vi "Startup.vi"(8 "error in (no error)":errorcluster, 11 "Data Cluster In":T1={"Status"="", "SQLite"=refnum, "StationConfig"={"station_id"="", "schema_version"="", "sqlite_path"="", "syncagent_db_path"="", "postgres_conn"="", "sync_interval_sec"=0, "inbound_offset_sec"=0, "batch_size"=0, "table_overrides"=[]}, "OB Module ID"=-1, "IB Module ID"=-1, "is online"=FALSE, "CM alive?"=FALSE, "OB alive?"=FALSE, "IB alive?"=FALSE, "IB first cycle seen?"=FALSE, "OB first cycle seen?"=FALSE, "shutting down?"=FALSE, "exit code"=0, "status"=FALSE, "code"=0, "source"="", "ShutdownReason"=enum."None", "OB last cycle at"=timestamp(0 s since 1904-01-01), "IB last cycle at"=timestamp(0 s since 1904-01-01), "Baseline Config"={"Baseline Mode"=enum."None", "From Date"="", "Chunk Size"=1000, "Verify Checksums"=TRUE}}) -> (0 "error out":errorcluster, 1 "halt?":bool, 3 "Data Cluster Out":T1={"Status"="", "SQLite"=refnum, "StationConfig"={"station_id"="", "schema_version"="", "sqlite_path"="", "syncagent_db_path"="", "postgres_conn"="", "sync_interval_sec"=0, "inbound_offset_sec"=0, "batch_size"=0, "table_overrides"=[]}, "OB Module ID"=-1, "IB Module ID"=-1, "is online"=FALSE, "CM alive?"=FALSE, "OB alive?"=FALSE, "IB alive?"=FALSE, "IB first cycle seen?"=FALSE, "OB first cycle seen?"=FALSE, "shutting down?"=FALSE, "exit code"=0, "status"=FALSE, "code"=0, "source"="", "ShutdownReason"=enum."None", "OB last cycle at"=timestamp(0 s since 1904-01-01), "IB last cycle at"=timestamp(0 s since 1904-01-01), "Baseline Config"={"Baseline Mode"=enum."None", "From Date"="", "Chunk Size"=1000, "Verify Checksums"=TRUE}})   [LabVIEW 2025, in "Dashboard.lvlib"]
uses:
  Dashboard.lvlib
  OpCore/SQLite/SQLite.lvclass
  OpCore/PostgreSQL/PostgreSQL.lvclass
  OpCore/Baseline/Baseline.lvclass
  OpCore/OpCore Foundation/OpCore Foundation.lvlib
  OpCore/OpCore Types/SyncCycleResult.ctl
  OpCore/OpCore Types/OpCore Types.lvlib
  OpCore/OpCore Types/CycleStatus.ctl
  OpCore/OpCore Types/CycleDirection.ctl
  OpCore/OpCore Types/SyncDirection.ctl
  OpCore/OpCore Types/TableOverride.ctl
  OpCore/OpCore Types/StationConfig.ctl
  OpCore/OpCore Types/ShutdownReason.ctl
  OpCore/OpCore Types/BaselineMode.ctl
  OpCore/OpCore Types/Baseline Config.ctl
  Module Data--cluster.ctl
panel:
  # "C:\\Works\\OpCore\\Data\\station-01.db"
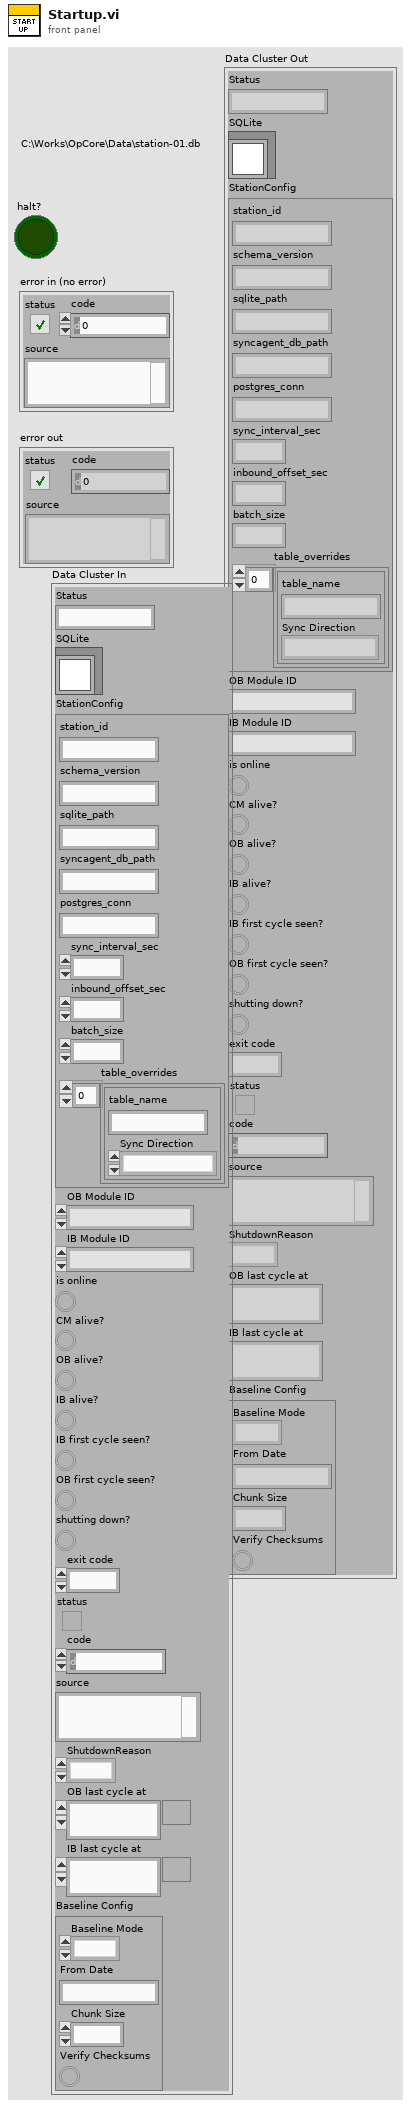
[diagram p1: front panel]
types:
  T1 = typedef "Dashboard.lvlib/Module Data--cluster.ctl" = cluster{"Status":string, "SQLite":refnum<class "SQLite.lvclass">, "StationConfig":T2, "OB Module ID":i32, "IB Module ID":i32, "is online":bool, "CM alive?":bool, "OB alive?":bool, "IB alive?":bool, "IB first cycle seen?":bool, "OB first cycle seen?":bool, "shutting down?":bool, "exit code":i32, "status":bool, "code":i32, "source":string, "ShutdownReason":T5, "OB last cycle at":timestamp, "IB last cycle at":timestamp, "Baseline Config":T6}
  T2 = typedef "OpCore Types.lvlib/StationConfig.ctl" = cluster{"station_id":string, "schema_version":string, "sqlite_path":string, "syncagent_db_path":string, "postgres_conn":string, "sync_interval_sec":i32, "inbound_offset_sec":i32, "batch_size":i32, "table_overrides":T3[]}
  T3 = typedef "OpCore Types.lvlib/TableOverride.ctl" = cluster{"table_name":string, "Sync Direction":T4}
  T4 = typedef "OpCore Types.lvlib/SyncDirection.ctl" = enum16{"Both", "Outbound_Only", "Inbound_Only", "Exclude"}
  T5 = typedef "OpCore Types.lvlib/ShutdownReason.ctl" = enum16{"None", "Operator", "Service", "ModuleDied", "Fatal"}
  T6 = typedef "OpCore Types.lvlib/Baseline Config.ctl" = cluster{"Baseline Mode":T7, "From Date":string, "Chunk Size":i32, "Verify Checksums":bool}
  T7 = typedef "OpCore Types.lvlib/BaselineMode.ctl" = enum16{"None", "Full", "From Date"}
  T8 = typedef "OpCore Types.lvlib/CycleStatus.ctl" = enum16{"Success", "Partial", "Failed"}
  T9 = typedef "OpCore Types.lvlib/CycleDirection.ctl" = enum16{"Outbound", "Inbound", "Startup", "Shutdown", "Baseline", "Provision", "Migration", "Config"}
  T10 = typedef "OpCore Types.lvlib/SyncCycleResult.ctl" = cluster{"Cycle Direction":T9, "records_synced":i32, "records_failed":i32, "Cycle Status":T8, "started_at":string, "finished_at":string, "error_detail":string}
  T11 = typedef "OpCore Types.lvlib/EnrolledTable.ctl" = cluster{"table_name":string, "uuid_column":string, "Sync Direction":T4, "is_enrolled":bool}
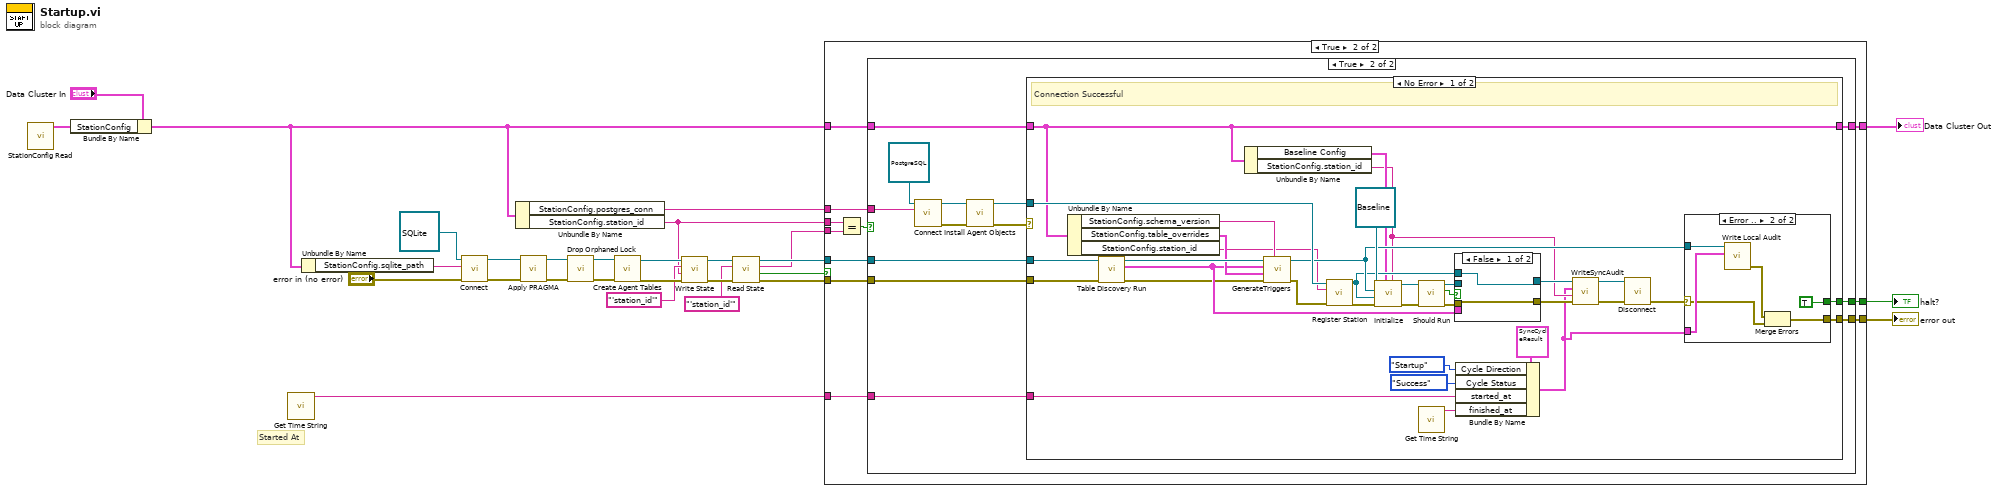
[diagram p0: block diagram]
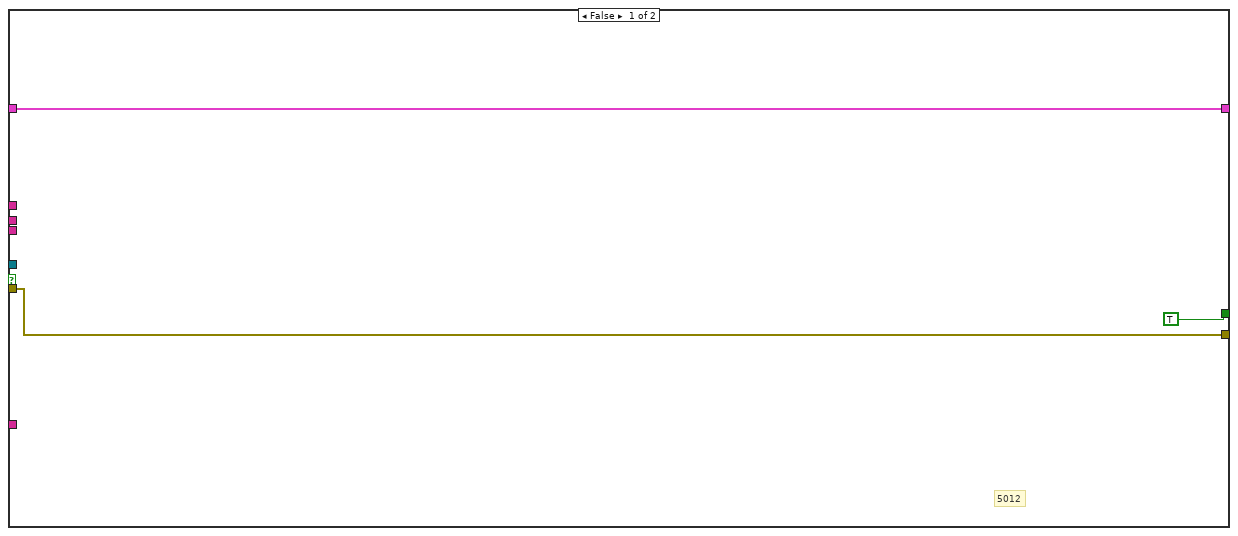
[diagram p2: hidden frame]
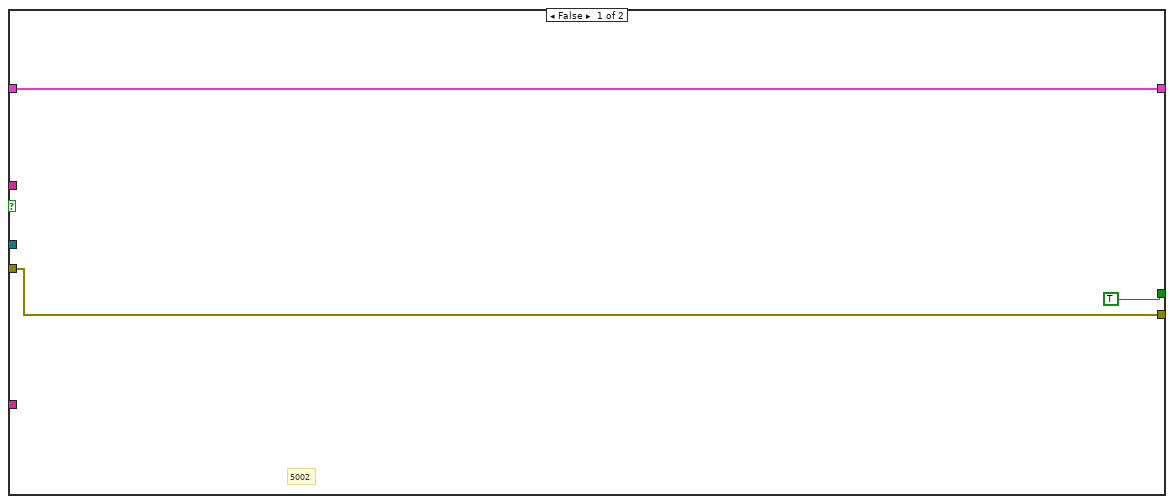
[diagram p3: hidden frame]
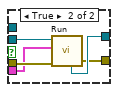
[diagram p4: hidden frame]
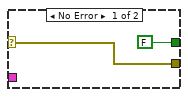
[diagram p5: hidden frame]
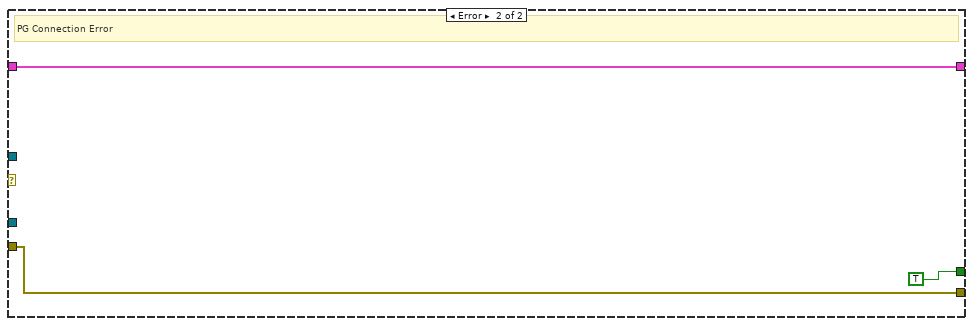
[diagram p6: hidden frame]
diagram:
  # "Started At"
  n1 = call "StationConfig Read.vi"() -> ("StationConfig"=w9:T2)  [unwired: 10 in, 1 out]
  n2 = Bundle By Name(cluster="Data Cluster In", "StationConfig"=w9) -> (w5:T1)
  n3 = call "Get Time String.vi"() -> ("Time String"=w20:string)  [unwired: 11 in]
  n4 = Unbundle By Name(w5) -> ("StationConfig.sqlite_path"=w4:string)
  n5 = call-dynamic "Connect.vi"("error in (no error)"="error in (no error)", "db_path"=w4, "SQLite in"=refnum<class "SQLite.lvclass"> refnum) -> ("error out"=w27:errorcluster, "SQLite out"=w28:refnum<class "SQLite.lvclass">)  [unwired: 7 in]
  n6 = Unbundle By Name(w5) -> ("StationConfig.postgres_conn"=w8:string, "StationConfig.station_id"=w6:string)
  n7 = call-dynamic "Apply PRAGMA.vi"("error in (no error)"=w27, "SQLite in"=w28) -> ("error out"=w25:errorcluster, "SQLite out"=w26:refnum<class "SQLite.lvclass">)  [unwired: 8 in]
  n8 = call "Drop Orphaned Lock.vi"("error in (no error)"=w25, "SQLite in"=w26) -> ("error out"=w24:errorcluster, "SQLite out"=w23:refnum<class "SQLite.lvclass">)  [unwired: 8 in]
  n9 = call "Create Agent Tables.vi"("error in (no error)"=w24, "SQLite in"=w23) -> ("error out"=w14:errorcluster, "SQLite out"=w13:refnum<class "SQLite.lvclass">)  [unwired: 8 in]
  n10 = call "Write State.vi"("error in (no error)"=w14, "Value"=w6, "Key"="'station_id'", "SQLite in"=w13) -> ("error out"=w11:errorcluster, "SQLite out"=w12:refnum<class "SQLite.lvclass">)  [unwired: 6 in]
  n11 = call "Read State.vi"("error in (no error)"=w11, "Key"="'station_id'", "SQLite in"=w12) -> ("error out"=w19:errorcluster, "Found?"=w22:bool, "Value"=w3:string, "SQLite out"=w21:refnum<class "SQLite.lvclass">)  [unwired: 5 in]
  n12 = case shown="True" w22 {
    tunnel: w21 -> [_ w41]
    tunnel: w20 -> [_ w40]
    tunnel: w19 -> [w30 w39]
    tunnel: [TRUE ("halt?") w38] -> w18
    tunnel: [w30 w37] -> w17
    tunnel: w5 -> [w29 w36]
    tunnel: [w29 w35] -> w2
    tunnel: w8 -> [_ w34]
    tunnel: w6 -> [_ w33]
    tunnel: w3 -> [_ w32]
    frame False {
      # "5012"
    }
    frame True {
      n13 = Equal?(x=w33, y=w32) -> (x = y?=w42:bool)
      n14 = case shown="True" w42 {
        tunnel: w41 -> [_ w58]
        tunnel: w40 -> [_ w57]
        tunnel: w39 -> [w44 w56]
        tunnel: [TRUE ("halt?") w55] -> w38
        tunnel: [w44 w54] -> w37
        tunnel: w36 -> [w43 w48]
        tunnel: [w43 w47] -> w35
        tunnel: w34 -> [_ w46]
        frame False {
          # "5002"
        }
        frame True {
          n15 = call-dynamic "Connect.vi"("Connection String"=w46, "PostgreSQL in"=refnum<class "PostgreSQL.lvclass"> refnum) -> ("error out"=w50:errorcluster, "PostgreSQL out"=w52:refnum<class "PostgreSQL.lvclass">)  [unwired: 8 in]
          n16 = call "Install Agent Objects.vi"("error in (no error)"=w50, "PostgreSQL in"=w52) -> ("error out"=w49:errorcluster, "PostgreSQL out"=w51:refnum<class "PostgreSQL.lvclass">)  [unwired: 8 in]
          n17 = case shown="No Error" w49 {
            tunnel: w58 -> [w77 _]
            tunnel: w51 -> [w93 _]
            tunnel: w57 -> [w64 _]
            tunnel: w56 -> [w79 w110]
            tunnel: [w87 TRUE ("halt?")] -> w55
            tunnel: [w86 w110] -> w54
            tunnel: w48 -> [w66 w109]
            tunnel: [w66 w109] -> w47
            frame No Error {
              # "Connection Successful"
              n18 = Unbundle By Name(w66) -> ("StationConfig.schema_version"=w75:string, "StationConfig.table_overrides"=w74:T3[], "StationConfig.station_id"=w59:string)
              n19 = call "Table Discovery Run.vi"("error in (no error)"=w79, "SQLite in"=w77) -> ("error out"=w72:errorcluster, "Enrolled Tables"=w73:T11[], "SQLite out"=w78:refnum<class "SQLite.lvclass">)  [unwired: 7 in]
              n20 = Unbundle By Name(w66) -> ("Baseline Config"=w67:T6, "StationConfig.station_id"=w65:string)
              n21 = call "GenerateTriggers.vi"("schema_version"=w75, "error in (no error)"=w72, "table_overrides"=w74, "enrolled_tables"=w73, "SQLite in"=w78) -> ("error out"=w88:errorcluster, "SQLite out"=w76:refnum<class "SQLite.lvclass">)  [unwired: 4 in, 1 out]
              n22 = call "Register Station.vi"("error in (no error)"=w88, "Station ID"=w59, "PostgreSQL in"=w93) -> ("error out"=w68:errorcluster, "PostgreSQL out"=w71:refnum<class "PostgreSQL.lvclass">)  [unwired: 7 in]
              n23 = call "Initialize.vi"("Station ID"=w65, "Baseline Config"=w67, "error in (no error)"=w68, "PostgreSQL.lvclass"=w71, "SQLite.lvclass"=w76, "Baseline in"=refnum<class "Baseline.lvclass"> refnum) -> ("error out"=w83:errorcluster, "Baseline out"=w84:refnum<class "Baseline.lvclass">)  [unwired: 4 in]
              n24 = call "Should Run.vi"("error in (no error)"=w83, "Baseline in"=w84) -> ("error out"=w81:errorcluster, "Should Run?"=w82:bool, "Baseline out"=w80:refnum<class "Baseline.lvclass">)  [unwired: 5 in, 2 out]
              n25 = call "Get Time String.vi"() -> ("Time String"=w89:string)  [unwired: 11 in]
              n26 = case shown="False" w82 {
                tunnel: w81 -> [w94 w100]
                tunnel: w80 -> [_ w99]
                tunnel: [w95 w98] -> w69
                tunnel: w71 -> [w95 _]
                tunnel: w73 -> [_ w97]
                tunnel: [w94 w96] -> w70
                frame False {
                }
                frame True {
                  n27 = call "Run.vi"("error in (no error)"=w100, "Enrolled Tables"=w97, "Baseline in"=w99) -> ("error out"=w96:errorcluster, "PostgreSQL"=w98:refnum<class "PostgreSQL.lvclass">)  [unwired: 4 in, 3 out]
                }
              }
              n28 = Bundle By Name(cluster=T10 {"Cycle Direction"=enum."Outbound", "records_synced"=0, "records_failed"=0, "Cycle Status"=enum."Success", "started_at"="", "finished_at"="", "error_detail"=""} ("SyncCycleResult"), "Cycle Direction"=CycleDirection."Startup", "Cycle Status"=CycleStatus."Success", "started_at"=w64, "finished_at"=w89) -> (w60:T10)
              n29 = call "WriteSyncAudit.vi"("error in (no error)"=w70, "station_id"=w65, "SyncCycleResult"=w60, "PostgreSQL in"=w69) -> ("error out"=w63:errorcluster, "PostgreSQL out"=w61:refnum<class "PostgreSQL.lvclass">)  [unwired: 6 in]
              n30 = call-dynamic "Disconnect.vi"("error in (no error)"=w63, "PostgreSQL in"=w61) -> ("error out"=w62:errorcluster)  [unwired: 9 in]
              n31 = case shown="Error .." w62 {
                selector: w62 -> [w101 w104]
                tunnel: [FALSE ("halt?") TRUE ("halt?")] -> w87
                tunnel: [w101 w103] -> w86
                tunnel: w76 -> [_ w107]
                tunnel: w60 -> [_ w106]
                frame No Error {
                }
                frame Error {
                  n32 = call "Write Local Audit.vi"("SyncCycleResult"=w106, "SQLite in"=w107) -> ("error out"=w105:errorcluster)  [unwired: 8 in, 1 out]
                  n33 = Merge Errors(w105, w104) -> (w103:errorcluster)
                }
              }
            }
            frame Error {
              # "PG Connection Error"
            }
          }
        }
      }
    }
  }
  "halt?" <- w18
  "error out" <- w17
  "Data Cluster Out" <- w2
